vi "SeriellReadFPGA.vi"   [LabVIEW 2010]
uses:
  <vilib>/eio/EIOMethodNode/EIOMethodNode.xnode
  <vilib>/rvi/DataTransferAndStorage/Container/XNode/niFpgaContainer.xnode
  <vilib>/rvi/DataTransferAndStorage/Container/Common/niFpgaTransferTypeControl.ctl
  <vilib>/rvi/DataTransferAndStorage/Container/Common/niFpgaContainerMethod.ctl
  <vilib>/rvi/interface/RandomDataEmulation/nirviRandomDataFPGAFIFO.vi
  <vilib>/rvi/interface/RandomDataEmulation/niFpgaRandomDataHandleErrors.vi
  markus/version feb 2012/gvboolesch.vi
types:
  T1 = typedef "niFpgaContainerMethod.ctl" = enum16{"<none>", "write", "read", "clear", "getNumberOfElementsToWrite", "getNumberOfElementsToRead", "enable", "disable", "flushAndDisable", "getStreamState", "readA", "readB", "dramWrite", "dramWriteWithByteEnables", "dramRequestData", "dramRetrieveData"}
  T2 = typedef "niFpgaTransferTypeControl.ctl" = enum16{"Target-Scoped", "Host to Target - DMA", "Target to Host - DMA", "Peer to Peer Reader", "Peer to Peer Writer", "Bidirectional"}
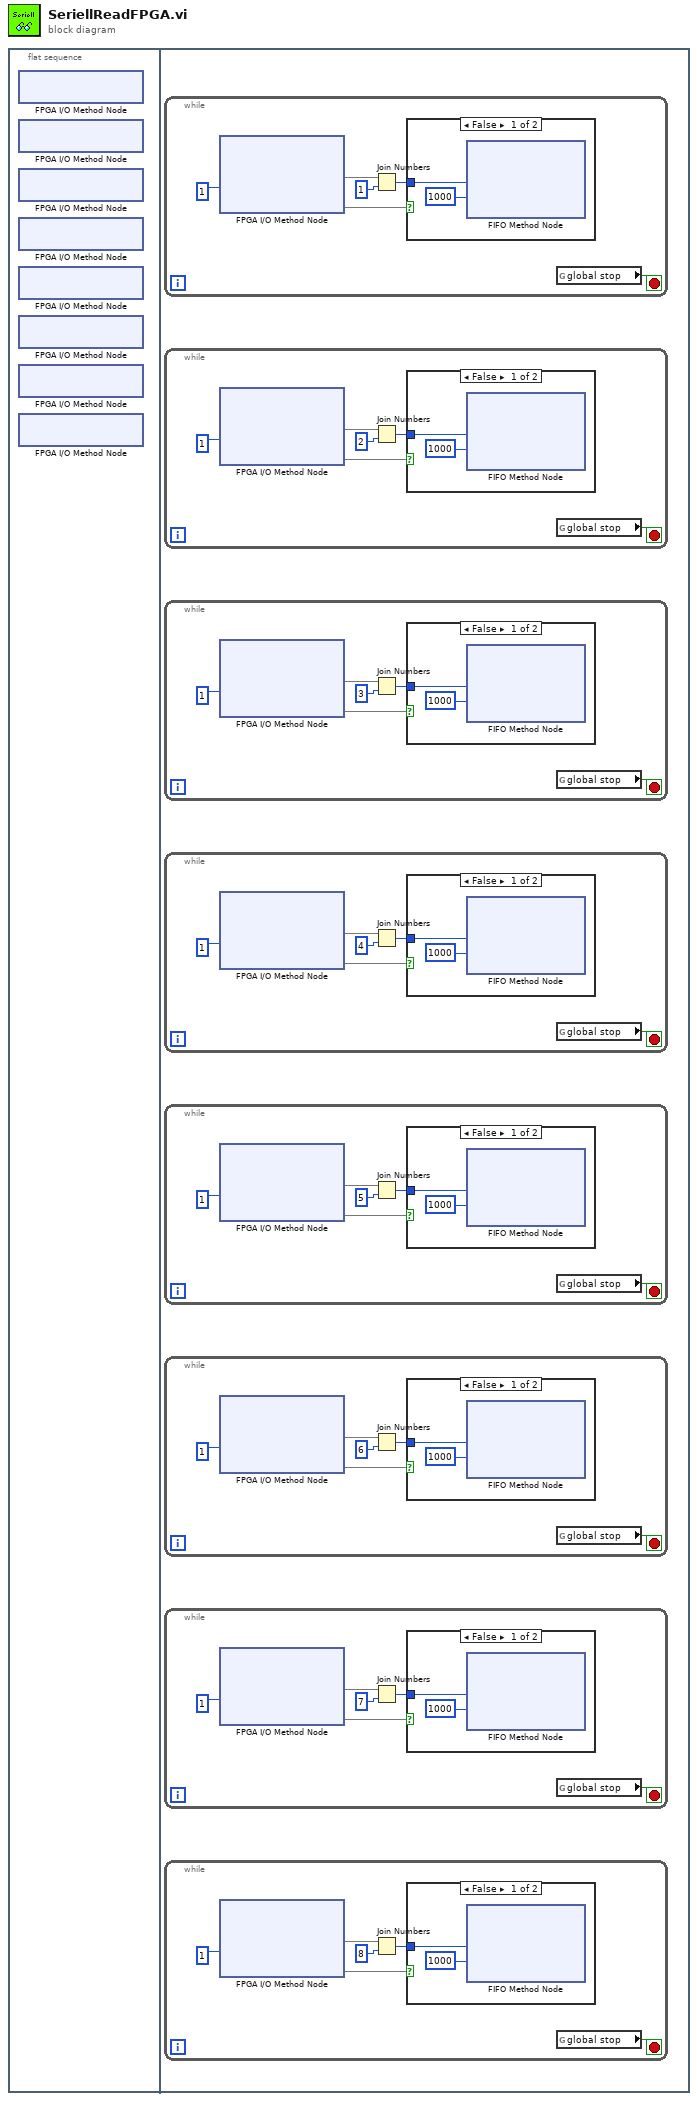
[diagram p0: block diagram]
diagram:
  n1 = flat-sequence {
    frame #0 {
      n2 = xnode "FPGA I/O Method Node"() -> ()  [unwired: 1 in, 1 out]
      n3 = xnode "FPGA I/O Method Node"() -> ()  [unwired: 1 in, 1 out]
      n4 = xnode "FPGA I/O Method Node"() -> ()  [unwired: 1 in, 1 out]
      n5 = xnode "FPGA I/O Method Node"() -> ()  [unwired: 1 in, 1 out]
      n6 = xnode "FPGA I/O Method Node"() -> ()  [unwired: 1 in, 1 out]
      n7 = xnode "FPGA I/O Method Node"() -> ()  [unwired: 1 in, 1 out]
      n8 = xnode "FPGA I/O Method Node"() -> ()  [unwired: 1 in, 1 out]
      n9 = xnode "FPGA I/O Method Node"() -> ()  [unwired: 1 in, 1 out]
    }
    frame #1 {
      n10 = while {
        stop <- w253 stop-if-true
        n11 = xnode "FPGA I/O Method Node"("Timeout (ms)"=1) -> ("Data"=w258, "Timed Out"=w256)  [unwired: 1 in, 1 out]
        n12 = Join Numbers(hi=w258, lo=u8 1) -> ((hi.lo)=w255:u16)
        n13 = case shown="False" w256 {
          tunnel: w255 -> [w260 _]
          frame False {
            n14 = xnode ("FIFO Method Node")("Element"=w260, "Timeout"=1000) -> ()  [unwired: 1 in, 2 out]
          }
          frame True {
          }
        }
        n15 = global read "gvboolesch.vi" "global stop"() -> (w253:bool)
      }
      n16 = while {
        stop <- w217 stop-if-true
        n17 = xnode "FPGA I/O Method Node"("Timeout (ms)"=1) -> ("Data"=w222, "Timed Out"=w220)  [unwired: 1 in, 1 out]
        n18 = Join Numbers(hi=w222, lo=u8 2) -> ((hi.lo)=w219:u16)
        n19 = case shown="False" w220 {
          tunnel: w219 -> [w224 _]
          frame False {
            n20 = xnode ("FIFO Method Node")("Element"=w224, "Timeout"=1000) -> ()  [unwired: 1 in, 2 out]
          }
          frame True {
          }
        }
        n21 = global read "gvboolesch.vi" "global stop"() -> (w217:bool)
      }
      n22 = while {
        stop <- w181 stop-if-true
        n23 = xnode "FPGA I/O Method Node"("Timeout (ms)"=1) -> ("Data"=w186, "Timed Out"=w184)  [unwired: 1 in, 1 out]
        n24 = Join Numbers(hi=w186, lo=u8 3) -> ((hi.lo)=w183:u16)
        n25 = case shown="False" w184 {
          tunnel: w183 -> [w188 _]
          frame False {
            n26 = xnode ("FIFO Method Node")("Element"=w188, "Timeout"=1000) -> ()  [unwired: 1 in, 2 out]
          }
          frame True {
          }
        }
        n27 = global read "gvboolesch.vi" "global stop"() -> (w181:bool)
      }
      n28 = while {
        stop <- w145 stop-if-true
        n29 = xnode "FPGA I/O Method Node"("Timeout (ms)"=1) -> ("Data"=w150, "Timed Out"=w148)  [unwired: 1 in, 1 out]
        n30 = Join Numbers(hi=w150, lo=u8 4) -> ((hi.lo)=w147:u16)
        n31 = case shown="False" w148 {
          tunnel: w147 -> [w152 _]
          frame False {
            n32 = xnode ("FIFO Method Node")("Element"=w152, "Timeout"=1000) -> ()  [unwired: 1 in, 2 out]
          }
          frame True {
          }
        }
        n33 = global read "gvboolesch.vi" "global stop"() -> (w145:bool)
      }
      n34 = while {
        stop <- w109 stop-if-true
        n35 = xnode "FPGA I/O Method Node"("Timeout (ms)"=1) -> ("Data"=w114, "Timed Out"=w112)  [unwired: 1 in, 1 out]
        n36 = Join Numbers(hi=w114, lo=u8 5) -> ((hi.lo)=w111:u16)
        n37 = case shown="False" w112 {
          tunnel: w111 -> [w116 _]
          frame False {
            n38 = xnode ("FIFO Method Node")("Element"=w116, "Timeout"=1000) -> ()  [unwired: 1 in, 2 out]
          }
          frame True {
          }
        }
        n39 = global read "gvboolesch.vi" "global stop"() -> (w109:bool)
      }
      n40 = while {
        stop <- w73 stop-if-true
        n41 = xnode "FPGA I/O Method Node"("Timeout (ms)"=1) -> ("Data"=w78, "Timed Out"=w76)  [unwired: 1 in, 1 out]
        n42 = Join Numbers(hi=w78, lo=u8 6) -> ((hi.lo)=w75:u16)
        n43 = case shown="False" w76 {
          tunnel: w75 -> [w80 _]
          frame False {
            n44 = xnode ("FIFO Method Node")("Element"=w80, "Timeout"=1000) -> ()  [unwired: 1 in, 2 out]
          }
          frame True {
          }
        }
        n45 = global read "gvboolesch.vi" "global stop"() -> (w73:bool)
      }
      n46 = while {
        stop <- w37 stop-if-true
        n47 = xnode "FPGA I/O Method Node"("Timeout (ms)"=1) -> ("Data"=w42, "Timed Out"=w40)  [unwired: 1 in, 1 out]
        n48 = Join Numbers(hi=w42, lo=u8 7) -> ((hi.lo)=w39:u16)
        n49 = case shown="False" w40 {
          tunnel: w39 -> [w44 _]
          frame False {
            n50 = xnode ("FIFO Method Node")("Element"=w44, "Timeout"=1000) -> ()  [unwired: 1 in, 2 out]
          }
          frame True {
          }
        }
        n51 = global read "gvboolesch.vi" "global stop"() -> (w37:bool)
      }
      n52 = while {
        stop <- w1 stop-if-true
        n53 = xnode "FPGA I/O Method Node"("Timeout (ms)"=1) -> ("Data"=w6, "Timed Out"=w4)  [unwired: 1 in, 1 out]
        n54 = Join Numbers(hi=w6, lo=u8 8) -> ((hi.lo)=w3:u16)
        n55 = case shown="False" w4 {
          tunnel: w3 -> [w8 _]
          frame False {
            n56 = xnode ("FIFO Method Node")("Element"=w8, "Timeout"=1000) -> ()  [unwired: 1 in, 2 out]
          }
          frame True {
          }
        }
        n57 = global read "gvboolesch.vi" "global stop"() -> (w1:bool)
      }
    }
  }
